vi "CompareIntegers.vi"(9 "Expected Value":i32, 10 "Actual Value":i32) -> (1 "Message":string, 2 "Equal?":bool)   [LabVIEW 2013, in "UnitTestComparisons.lvlib"]
uses:
  UnitTestComparisons.lvlib
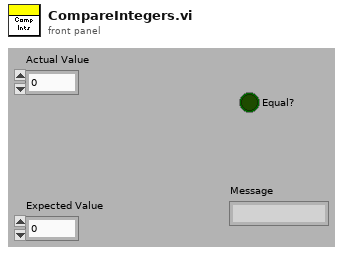
[diagram p1: front panel]
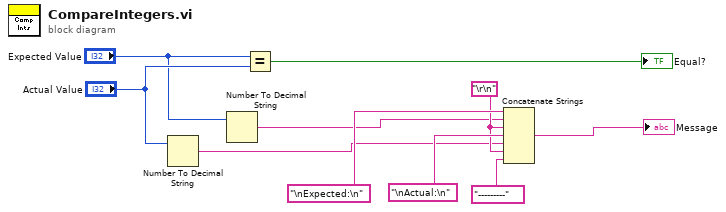
[diagram p0: block diagram]
diagram:
  w4 = "\r\n"
  n1 = Number To Decimal String(number="Actual Value") -> (decimal integer string=w1:string)  [unwired: 1 in]
  n2 = Number To Decimal String(number="Expected Value") -> (decimal integer string=w2:string)  [unwired: 1 in]
  n3 = Equal?(x="Expected Value", y="Actual Value") -> (x = y?=→"Equal?":bool)
  n4 = Concatenate Strings("\nExpected:\n" ("string"), w2, w4, "\nActual:\n" ("string"), w1, w4, "---------" ("string")) -> (→"Message":string)
